vi "Bloomy Battery Simulator 1200 VI Tree.vi"   [LabVIEW 2021]
doc: "This is the VI tree for the Bloomy Battery Simulator 1200, showing how the driver should be used to control the instrument."
uses:
  BS120x Driver.lvlib
  BS120x.lvclass
  Public/New BS120x Device/New BS120x Ethernet Device.vi
panel:
  # "See Diagram\nFor VI Tree"
  # "(c) 2024 Bloomy Controls, Inc. All rights reserved."
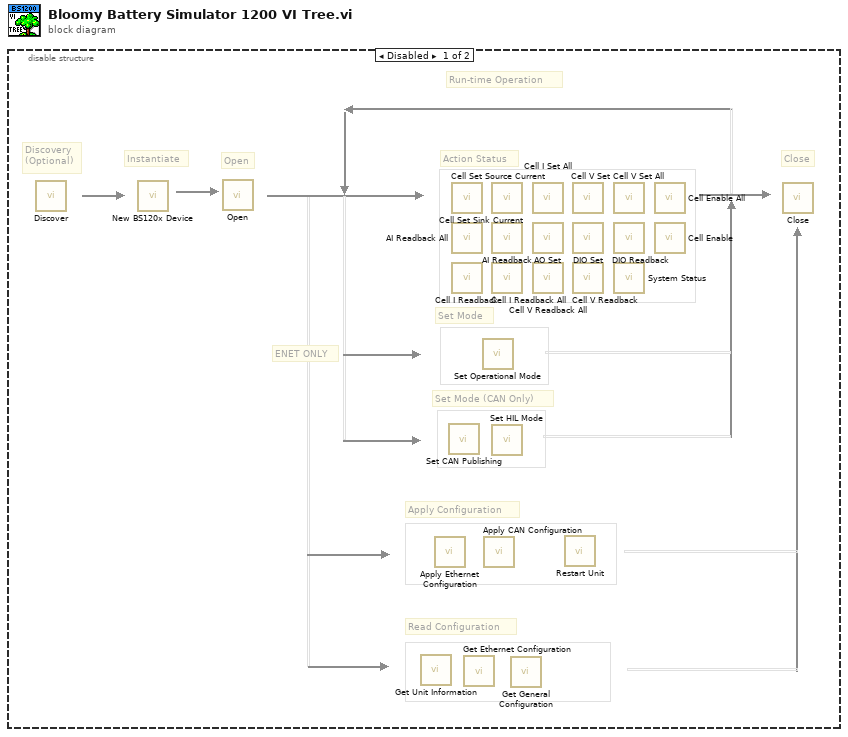
[diagram p0: block diagram]
diagram:
  n1 = disable-structure shown="Disabled" {
    frame Disabled {
      # "Open"
      # "Discovery\n(Optional)"
      # "ENET ONLY"
      # "Set Mode (CAN Only)"
      # "Run-time Operation"
      # "Read Configuration"
      # "Apply Configuration"
      # "Close"
      # "Action Status"
      # "Set Mode"
      # "Instantiate"
      n2 = call "Discover.vi"() -> ()  [unwired: 10 in, 2 out]
      n3 = call-poly "New BS120x Device.vi"() -> ()  [unwired: 10 in, 2 out]
      n4 = call-dynamic "Open.vi"() -> ()  [unwired: 10 in, 2 out]
      n5 = call-dynamic "Get Unit Information.vi"() -> ()  [unwired: 7 in, 5 out]
      n6 = call-dynamic "Apply Ethernet Configuration.vi"() -> ()  [unwired: 10 in, 2 out]
      n7 = call-dynamic "Set CAN Publishing.vi"() -> ()  [unwired: 10 in, 2 out]
      n8 = call-dynamic "Cell Set Source Current.vi"() -> ()  [unwired: 10 in, 2 out]
      n9 = call-dynamic "AI Readback All.vi"() -> ()  [unwired: 9 in, 3 out]
      n10 = call-dynamic "Cell I Readback.vi"() -> ()  [unwired: 9 in, 3 out]
      n11 = call-dynamic "Get Ethernet Configuration.vi"() -> ()  [unwired: 8 in, 4 out]
      n12 = call-dynamic "Set Operational Mode.vi"() -> ()  [unwired: 10 in, 2 out]
      n13 = call-dynamic "Apply CAN Configuration.vi"() -> ()  [unwired: 10 in, 2 out]
      n14 = call-dynamic "Cell Set Sink Current.vi"() -> ()  [unwired: 10 in, 2 out]
      n15 = call-dynamic "AI Readback.vi"() -> ()  [unwired: 9 in, 3 out]
      n16 = call-dynamic "Cell I Readback All.vi"() -> ()  [unwired: 9 in, 3 out]
      n17 = call-dynamic "Set HIL Mode.vi"() -> ()  [unwired: 10 in, 2 out]
      n18 = call-dynamic "Get General Configuration.vi"() -> ()  [unwired: 7 in, 5 out]
      n19 = call-dynamic "Cell I Set All.vi"() -> ()  [unwired: 10 in, 2 out]
      n20 = call-dynamic "AO Set.vi"() -> ()  [unwired: 10 in, 2 out]
      n21 = call-dynamic "Cell V Readback All.vi"() -> ()  [unwired: 9 in, 3 out]
      n22 = call-dynamic "Restart Unit.vi"() -> ()  [unwired: 10 in, 2 out]
      n23 = call-dynamic "Cell V Set.vi"() -> ()  [unwired: 10 in, 2 out]
      n24 = call-dynamic "DIO Set.vi"() -> ()  [unwired: 10 in, 2 out]
      n25 = call-dynamic "Cell V Readback.vi"() -> ()  [unwired: 9 in, 3 out]
      n26 = call-dynamic "Cell V Set All.vi"() -> ()  [unwired: 10 in, 2 out]
      n27 = call-dynamic "DIO Readback.vi"() -> ()  [unwired: 9 in, 3 out]
      n28 = call-dynamic "System Status.vi"() -> ()  [unwired: 9 in, 3 out]
      n29 = call-dynamic "Cell Enable All.vi"() -> ()  [unwired: 10 in, 2 out]
      n30 = call-dynamic "Cell Enable.vi"() -> ()  [unwired: 10 in, 2 out]
      n31 = call-dynamic "Close.vi"() -> ()  [unwired: 10 in, 2 out]
    }
    frame Enabled {
    }
  }
